vi "Drift Correct Scan Frame.vi"(6 "Scan Parameters in":T1 {"Avoid zero threshold (V)" format="%#_13g"}, 9 "ScanQ in":refnum<queue>, 10 "Dx, Dy":cluster{"Xc":sgl, "Yc":sgl}={"Xc"=nan, "Yc"=nan} caption="Drift  (m) (NaN=no change)" {"Yc" format="%.2p"; "Xc" format="%.2p"}, 11 "Queue in":refnum<queue>) -> (0 "error out":errorcluster, 1 "return value":cluster{"x":dbl, "y":dbl}, 2 "Scan Parameters out":T1 {"Avoid zero threshold (V)" format="%#_13g"}, 3 "Queue out":refnum<queue>, 5 "Corrected Coordinates":cluster{"Initial x":dbl, "Initial y":dbl}, 7 "ScanQ out":refnum<queue>)   [LabVIEW 2025]
uses:
  CTLS/ACK.ctl
  <userlib>/Nanonis Prog Interface V5e/Nanonis Prog Interface.lvlib
  CTLS/Scan_Params (QMH).ctl
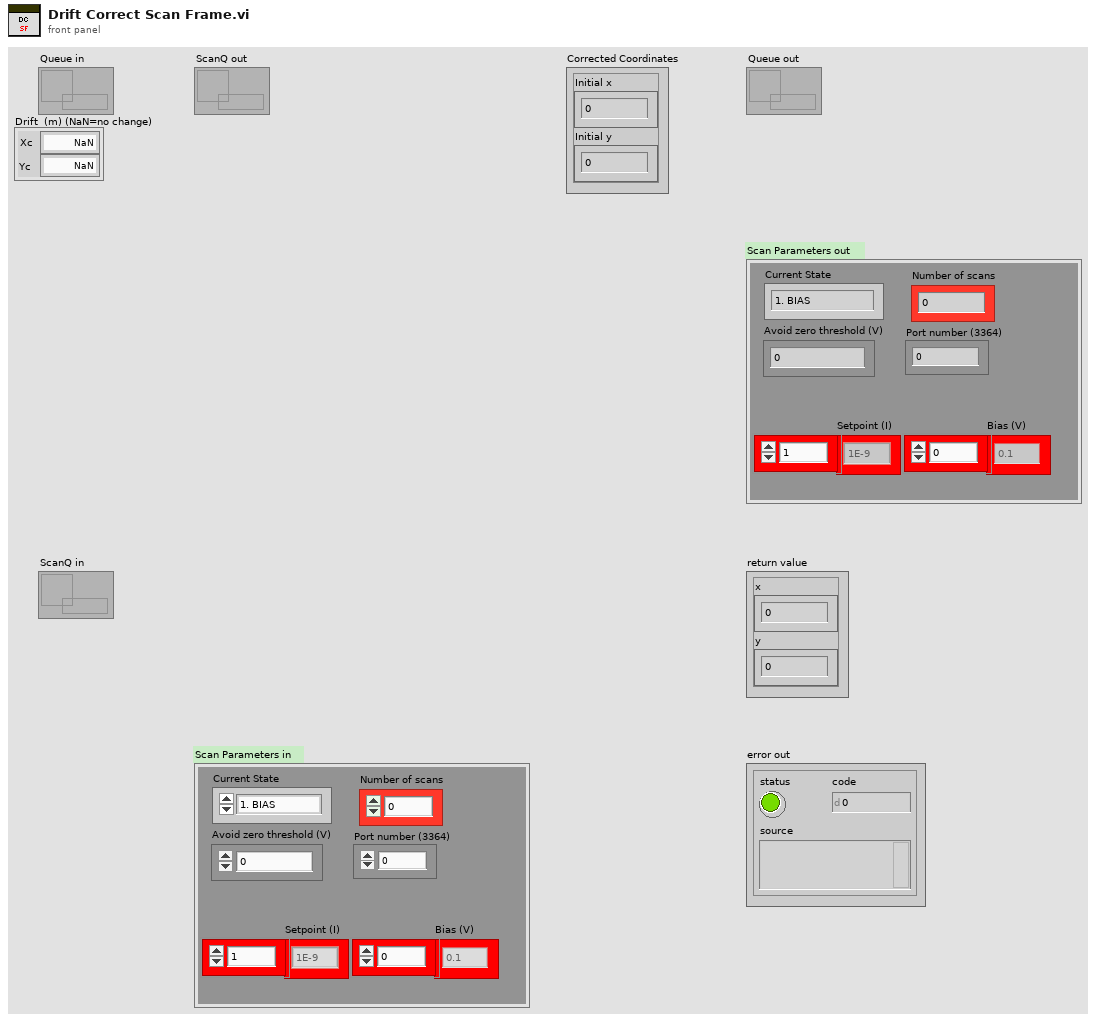
[diagram p1: front panel]
types:
  T1 = typedef "Scan_Params (QMH).ctl" = cluster{"Setpoint (I)":dbl[], "Bias (V)":dbl[], "Number of scans":u8, "Port number (3364)":u32, "Avoid zero threshold (V)":dbl, "Current State":enum16{"1. BIAS", "2. POLL BIAS", "3. SCAN", "4. SCAN_IDLE", "5. Drift_Correct (SF)", "6. Drift_Correct (BS)", "7. STOP"}}
  T2 = enum16{"1. None", "2. TempStable", "3. FieldStable", "4. ConfigApplied", "5. ScanDone", "6. BiasDone", "7. DriftDone (SF)", "8. DrifDone (BS)"}
  T3 = typedef "ACK.ctl" = cluster{"ACK":enum16{"1. None", "2. TempStable", "3. FieldStable", "4. ConfigApplied", "5. ScanDone", "6. BiasDone", "7. DriftDone (SF)", "8. DrifDone (BS)"}}
  T4 = enum16{"1. BIAS", "2. POLL BIAS", "3. SCAN", "4. SCAN_IDLE", "5. Drift_Correct (SF)", "6. Drift_Correct (BS)", "7. STOP"}
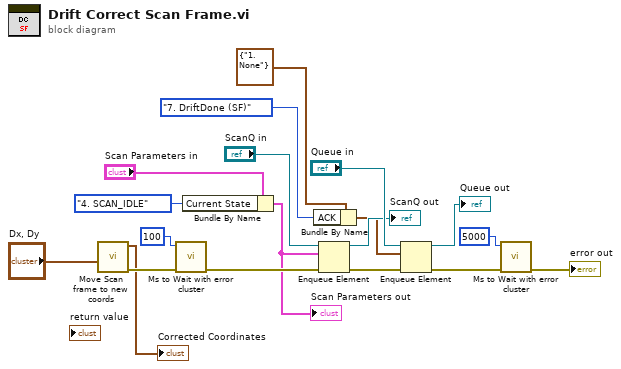
[diagram p0: block diagram]
diagram:
  n1 = call "Move Scan frame to new coords.vi"("Dx, Dy"="Dx, Dy") -> ("Corrected Coordinates"=→"Corrected Coordinates":cluster{"Initial x":dbl, "Initial y":dbl}, "error out"=w17:errorcluster)  [unwired: 8 in]
  n2 = call <userlib>:"Ms to Wait with error cluster.vi"("error in (no error)"=w17, "milliseconds to wait"=u32 100) -> ("error out"=w18:errorcluster)  [unwired: 4 in, 1 out]
  n3 = Bundle By Name(cluster="Scan Parameters in", "Current State"=T4."4. SCAN_IDLE") -> (w12:T1)
  "Scan Parameters out" <- w12
  n4 = Bundle By Name(cluster=T3 {"ACK"=enum."1. None"} ("Acknowledements"), "ACK"=T2."7. DriftDone (SF)") -> (w3:T3)
  n5 = Enqueue Element(queue="ScanQ in", element=w12, error in (no error)=w18) -> (queue out=→"ScanQ out":refnum<queue>, error out=w4:errorcluster)  [unwired: 1 in, 1 out]
  n6 = Enqueue Element(queue="Queue in", element=w3, error in (no error)=w4) -> (queue out=→"Queue out":refnum<queue>, error out=w13:errorcluster)  [unwired: 1 in, 1 out]
  n7 = call <userlib>:"Ms to Wait with error cluster.vi"("error in (no error)"=w13, "milliseconds to wait"=u32 5000) -> ("error out"=→"error out":errorcluster)  [unwired: 4 in, 1 out]
